vi "Init Prefs.vi"(8 "error in (no error)":errorcluster, 11 "GUI Helper in":refnum<class "GUI Helper.lvclass">) -> (0 "error out":errorcluster, 3 "GUI Helper out":refnum<class "GUI Helper.lvclass">)   [LabVIEW 2020, in "VolatusGUI.lvlib" / "GUI Helper.lvclass"]
uses:
  GUI Helper.lvclass
  GUIStateValue/GUIStateValue.lvclass
  GUI Helper.lvclass/GUI Helper.ctl
  Volatus/MessageQ/MessageQ.lvclass
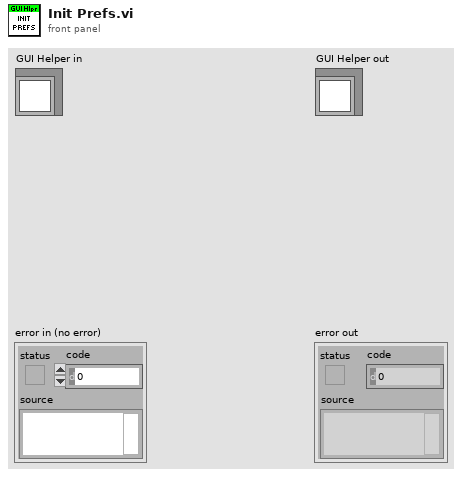
[diagram p1: front panel]
types:
  T1 = typedef "VolatusGUI.lvlib/GUI State.ctl" = cluster{"GUI ID":string, "Visible":bool, "Visibility Set":bool, "Bounds":T2, "Bounds Set":bool}
  T2 = typedef "LVRectTypeDef.ctl" = cluster{"Left":i16, "Top":i16, "Right":i16, "Bottom":i16}
  T3 = enum32{"Invalid", "Standard", "Closed", "Hidden", "Minimized", "Maximized"}
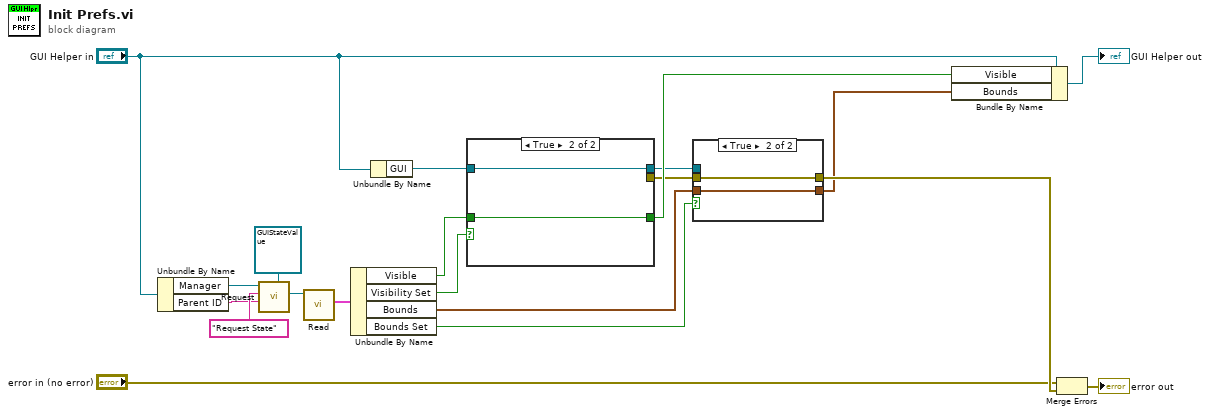
[diagram p0: block diagram]
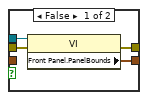
[diagram p2: hidden frame]
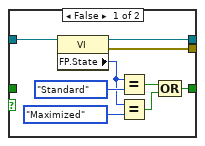
[diagram p3: hidden frame]
diagram:
  n1 = Unbundle By Name("GUI Helper in") -> ("Manager"=w15:refnum<class "MessageQ.lvclass">, "Parent ID"=w1:string)
  n2 = call "Request.vi"("Response Type (None)"=refnum<class "GUIStateValue.lvclass"> refnum ("VolatusGUI:GUIStateValue.lvclass"), "Data"=w1, "ID"="Request State", "MessageQ in"=w15) -> ("Response"=w16:refnum<class "GUIStateValue.lvclass">)  [unwired: 5 in, 2 out]
  n3 = call "Read.vi"("GUIStateValue in"=w16) -> ("GUI State"=w14:T1)  [unwired: 10 in]
  n4 = Unbundle By Name(w14) -> ("Visible"=w11:bool, "Visibility Set"=w12:bool, "Bounds"=w7:T2, "Bounds Set"=w6:bool)
  n5 = Unbundle By Name("GUI Helper in") -> ("GUI"=w10:refnum<vi>)
  n6 = case shown="True" w12 {
    tunnel: w11 -> [_ w31]
    tunnel: w10 -> [w29 w30]
    tunnel: [w23 w31] -> w9
    tunnel: [w22 w30] -> w8
    tunnel: [w21 _] -> w4
    frame False {
      n7 = property class="VI"(reference=w29) -> (reference out=w22:refnum<vi>, error out=w21:errorcluster, "FP.State"=w26:T3)  [unwired: 1 in]
      n8 = Equal?(x=w26, y=T3."Standard") -> (x = y?=w25:bool)
      n9 = Equal?(x=w26, y=T3."Maximized") -> (x = y?=w24:bool)
      n10 = Compound Arithmetic op=OR(w25, w24) -> (w23:bool)
    }
    frame True {
    }
  }
  n11 = case shown="True" w6 {
    tunnel: w8 -> [w35 _]
    tunnel: w7 -> [_ w37]
    tunnel: [w34 w37] -> w5
    tunnel: w4 -> [w33 w36]
    tunnel: [w32 w36] -> w20
    frame False {
      n12 = property class="VI"(reference=w35, error in=w33) -> (error out=w32:errorcluster, "Front Panel.PanelBounds"=w34:T2)  [unwired: 1 out]
    }
    frame True {
    }
  }
  n13 = Bundle By Name(cluster="GUI Helper in", "Visible"=w9, "Bounds"=w5) -> (→"GUI Helper out":refnum<class "GUI Helper.lvclass">)
  n14 = Merge Errors("error in (no error)", w20) -> (→"error out":errorcluster)
